vi "savenload.vi"() -> (3 "load error":bool)   [LabVIEW 2012]
uses:
  G_DATA.vi
  G_VEH.vi
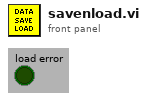
[diagram p1: front panel]
types:
  T1 = enum16{"open", "replace", "create", "open or create", "replace or create", "replace or create with confirmation"}
  T2 = cluster{"M6006":string, "M7042":string, "Tcandata":string, "LaserData":string, "SensorData":string, "B_Sencor data 2202":string, "B_object data 2221":string, "Tmobileye":string}
  T3 = cluster{"M6006":string, "M7042":string, "Tcandata":string, "LaserData":string, "SensorData":string, "B_Sencor data 2202":string, "B_object data 2221":string}
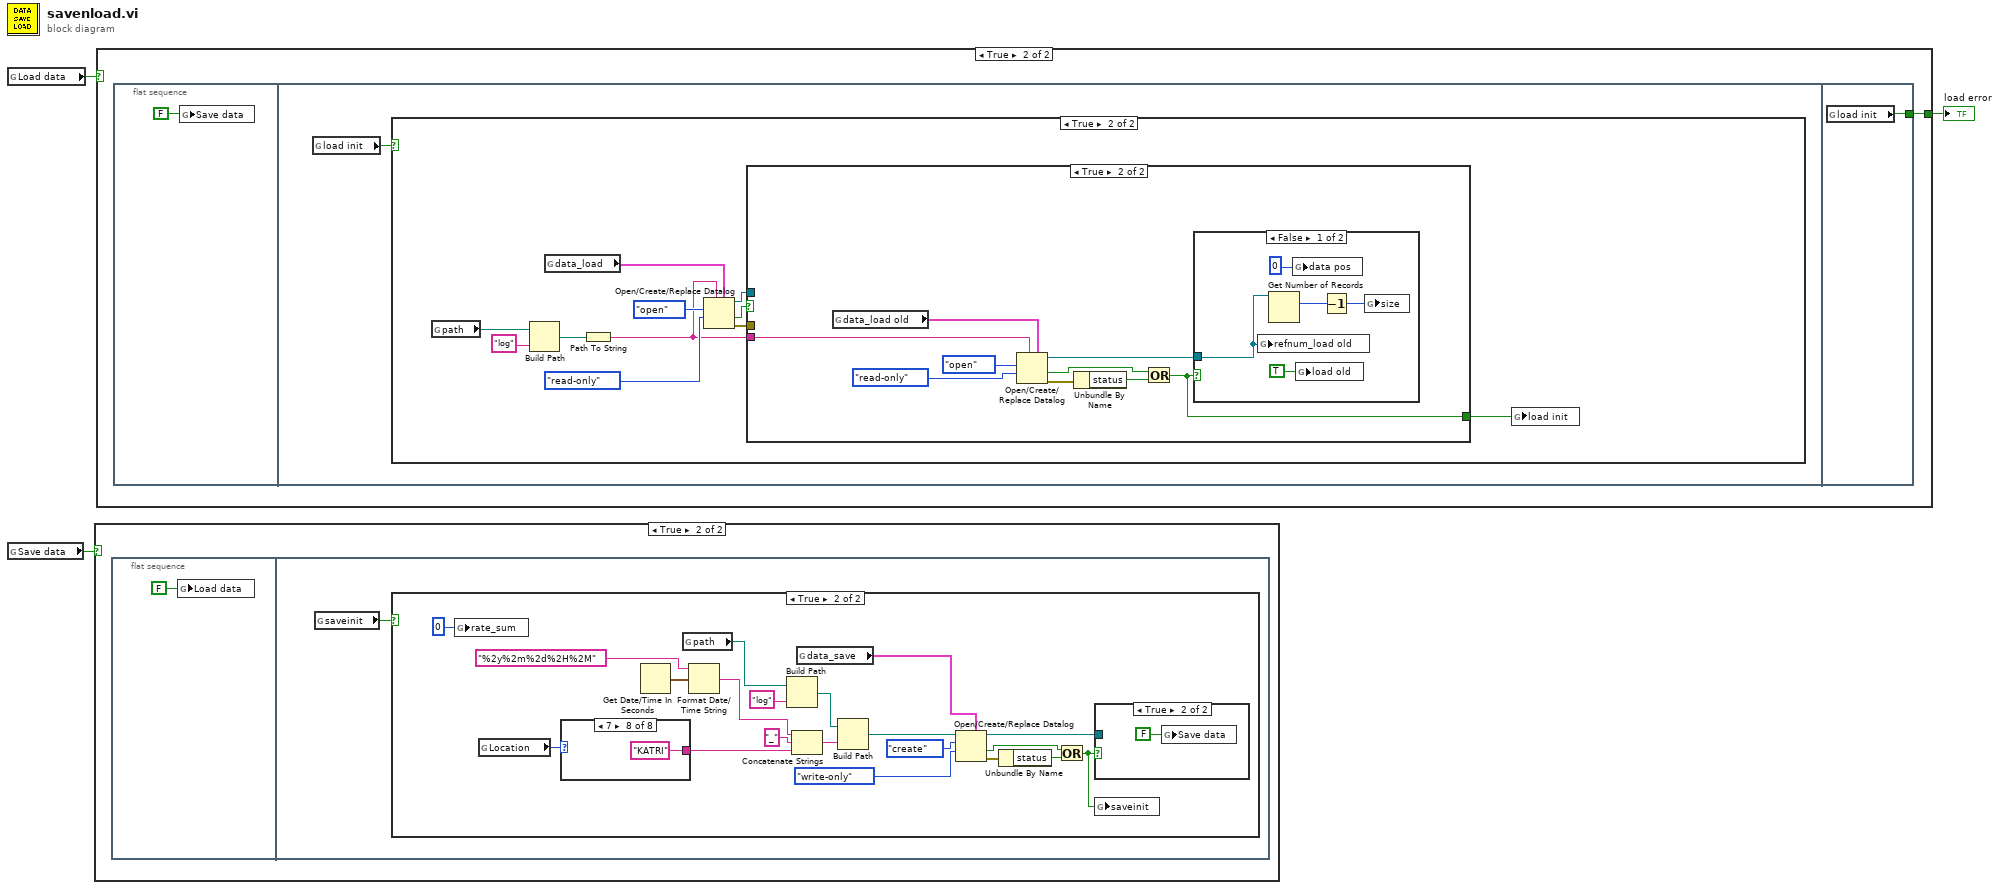
[diagram p0: block diagram]
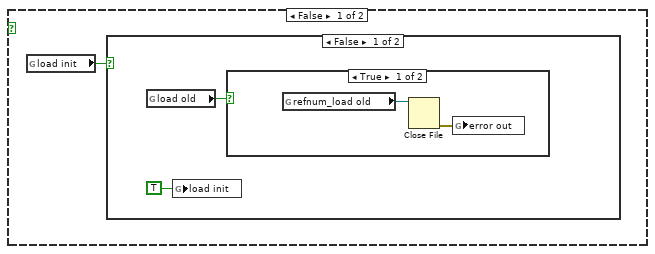
[diagram p2: hidden frame]
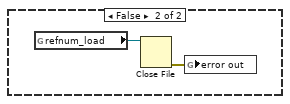
[diagram p3: hidden frame]
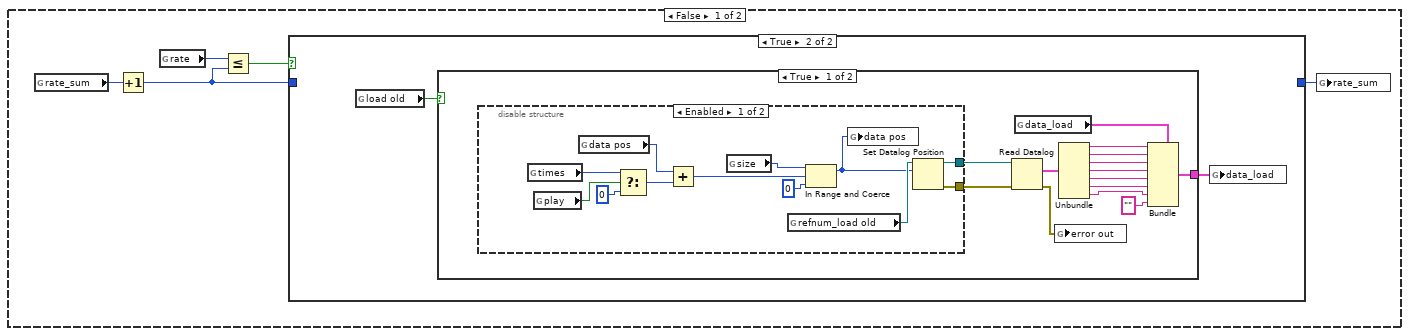
[diagram p5: hidden frame]
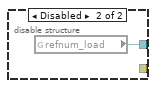
[diagram p7: hidden frame]
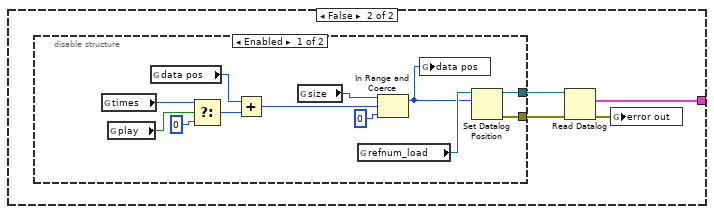
[diagram p8: hidden frame]
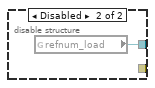
[diagram p9: hidden frame]
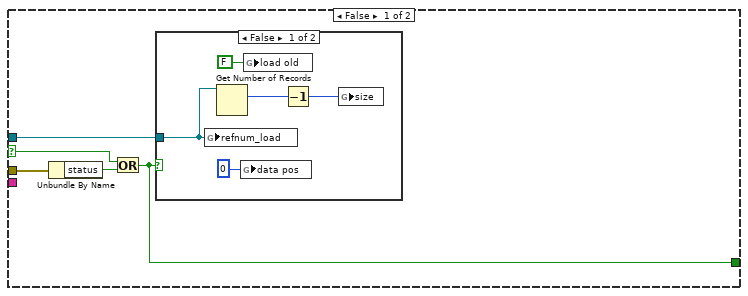
[diagram p10: hidden frame]
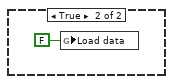
[diagram p11: hidden frame]
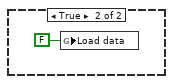
[diagram p12: hidden frame]
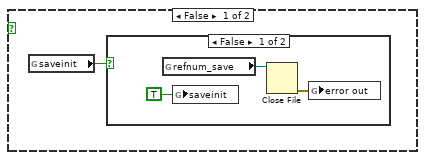
[diagram p13: hidden frame]
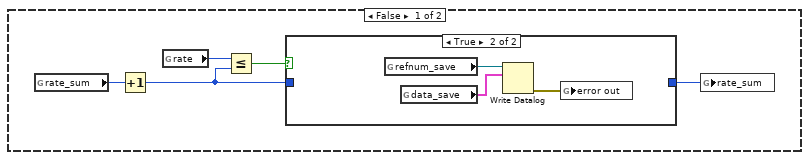
[diagram p15: hidden frame]
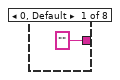
[diagram p17: hidden frame]
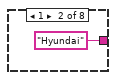
[diagram p18: hidden frame]
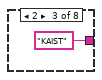
[diagram p19: hidden frame]
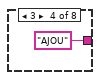
[diagram p20: hidden frame]
diagram:
  n1 = global read "G_DATA.vi" "Load data"() -> (w1:bool)
  n2 = global read "G_DATA.vi" "Save data"() -> (w3:bool)
  n3 = case shown="True" w3 {
    frame False {
      n4 = global read "G_DATA.vi" "saveinit"() -> (w4:bool)
      n5 = case shown="False" w4 {
        frame False {
          n6 = global read "G_DATA.vi" "refnum_save"() -> (w7:refnum<k1>)
          n7 = global write "G_DATA.vi" "saveinit"(TRUE ("saveinit")) -> ()
          n8 = Close File(refnum=w7) -> (error out=w5:errorcluster)  [unwired: 1 in, 1 out]
          n9 = global write "G_DATA.vi" "error out"(w5) -> ()
        }
        frame True {
        }
      }
    }
    frame True {
      n10 = flat-sequence {
        frame #0 {
          n11 = global write "G_DATA.vi" "Load data"(FALSE ("Visible")) -> ()
        }
        frame #1 {
          n12 = global read "G_DATA.vi" "saveinit"() -> (w9:bool)
          n13 = case shown="True" w9 {
            frame False {
              n14 = global read "G_DATA.vi" "rate_sum"() -> (w14:u8)
              n15 = Increment(x=w14) -> (x+1=w10:u8)
              n16 = global read "G_DATA.vi" "rate"() -> (w11:u8)
              n17 = Less Or Equal?(x=w11, y=w10) -> (x <= y?=w13:bool)
              n18 = case shown="True" w13 {
                tunnel: [w15 _] -> w12
                tunnel: w10 -> [w15 _]
                frame False {
                }
                frame True {
                  n19 = global read "G_DATA.vi" "refnum_save"() -> (w18:refnum<k1>)
                  n20 = global read "G_DATA.vi" "data_save"() -> (w17:T2)
                  n21 = Write Datalog(6:w17, 7:w18) -> (0:w16:errorcluster)  [unwired: 1 in, 1 out]
                  n22 = global write "G_DATA.vi" "error out"(w16) -> ()
                }
              }
              n23 = global write "G_DATA.vi" "rate_sum"(w12) -> ()
            }
            frame True {
              n24 = global write "G_DATA.vi" "rate_sum"(u8 0 ("rate_sum")) -> ()
              n25 = global read "G_VEH.vi" "Location"() -> (w29:i32)
              n26 = case shown="7" w29 {
                tunnel: ["" ("String") "Hyundai" ("String") "KAIST" ("String") "AJOU" ("String") "MUNJI" ("String") "Airforce" ("String") "CAR" ("String") "KATRI" ("String")] -> w28
                frame 0, Default {
                }
                frame 1 {
                }
                frame 2 {
                }
                frame 3 {
                }
                frame 4 {
                }
                frame 5 {
                }
                frame 6 {
                }
                frame 7 {
                }
              }
              n27 = Get Date/Time In Seconds() -> (seconds since 1Jan1904=w32:timestamp)
              n28 = global read "G_DATA.vi" "path"() -> (w20:path)
              n29 = Format Date/Time String(time format string (%c)="%2y%2m%2d%2H%2M", seconds (now)=w32) -> (date/time string=w26:string)  [unwired: 1 in]
              n30 = Build Path(base path=w20, name or relative path="log") -> (appended path=w19:path)
              n31 = Concatenate Strings(w26, "_" ("string"), w28) -> (w25:string)
              n32 = global read "G_DATA.vi" "data_save"() -> (w35:T2)
              n33 = Build Path(base path=w19, name or relative path=w25) -> (appended path=w30:path)
              n34 = Open/Create/Replace Datalog(5:w35, 9:enum16{"read/write", "read-only", "write-only"}."write-only" ("access (0:read/write)"), 10:T1."create" ("operation (0:open)"), 11:w30) -> (0:w36:errorcluster, 1:w24:bool, 3:w34:refnum<k1>)  [unwired: 1 in, 1 out]
              n35 = Unbundle By Name(w36) -> ("status"=w23:bool)
              n36 = Or(x=w24, y=w23) -> (x .or. y?=w22:bool)
              n37 = case shown="True" w22 {
                tunnel: w34 -> [w47 _]
                frame False {
                  n38 = global write "G_DATA.vi" "refnum_save"(w47) -> ()
                }
                frame True {
                  n39 = global write "G_DATA.vi" "Save data"(FALSE ("Save data")) -> ()
                }
              }
              n40 = global write "G_DATA.vi" "saveinit"(w22) -> ()
            }
          }
        }
      }
    }
  }
  n41 = case shown="True" w1 {
    tunnel: [_ w56] -> w2
    frame False {
      n42 = global read "G_DATA.vi" "load init"() -> (w49:bool)
      n43 = case shown="False" w49 {
        frame False {
          n44 = global read "G_DATA.vi" "load old"() -> (w50:bool)
          n45 = global write "G_DATA.vi" "load init"(TRUE ("saveinit")) -> ()
          n46 = case shown="True" w50 {
            frame True {
              n47 = global read "G_DATA.vi" "refnum_load old"() -> (w52:refnum<k1>)
              n48 = Close File(refnum=w52) -> (error out=w53:errorcluster)  [unwired: 1 in, 1 out]
              n49 = global write "G_DATA.vi" "error out"(w53) -> ()
            }
            frame False {
              n50 = global read "G_DATA.vi" "refnum_load"() -> (w54:refnum<k1>)
              n51 = Close File(refnum=w54) -> (error out=w55:errorcluster)  [unwired: 1 in, 1 out]
              n52 = global write "G_DATA.vi" "error out"(w55) -> ()
            }
          }
        }
        frame True {
        }
      }
    }
    frame True {
      n53 = flat-sequence {
        tunnel: [w148] -> w56
        frame #0 {
          n54 = global write "G_DATA.vi" "Save data"(FALSE ("Save data")) -> ()
        }
        frame #1 {
          n55 = global read "G_DATA.vi" "load init"() -> (w58:bool)
          n56 = case shown="True" w58 {
            frame False {
              n57 = global read "G_DATA.vi" "rate_sum"() -> (w62:u8)
              n58 = Increment(x=w62) -> (x+1=w59:u8)
              n59 = global read "G_DATA.vi" "rate"() -> (w63:u8)
              n60 = Less Or Equal?(x=w63, y=w59) -> (x <= y?=w61:bool)
              n61 = case shown="True" w61 {
                tunnel: [w64 _] -> w60
                tunnel: w59 -> [w64 _]
                frame False {
                }
                frame True {
                  n62 = global read "G_DATA.vi" "load old"() -> (w66:bool)
                  n63 = case shown="True" w66 {
                    tunnel: [w70 w94] -> w65
                    frame True {
                      n64 = disable-structure shown="Enabled" {
                        disable-tunnel: [w84 _] -> w80
                        disable-tunnel: [w83 w93] -> w78
                        frame Enabled {
                          n65 = global read "G_DATA.vi" "times"() -> (w89:i64)
                          n66 = global read "G_DATA.vi" "play"() -> (w90:bool)
                          n67 = global read "G_DATA.vi" "data pos"() -> (w92:i64)
                          n68 = Select(t=w89, s=w90, f=i64 0) -> (s? t:f=w85:i64)
                          n69 = Add(x=w92, y=w85) -> (x+y=w87:i64)
                          n70 = global read "G_DATA.vi" "size"() -> (w91:i64)
                          n71 = global read "G_DATA.vi" "refnum_load old"() -> (w82:refnum<k1>)
                          n72 = In Range and Coerce(upper limit=w91, x=w87, lower limit=i64 0) -> (coerced(x)=w81:i64)  [unwired: 1 out]
                          n73 = global write "G_DATA.vi" "data pos"(w81) -> ()
                          n74 = Set Datalog Position(6:w81, 7:w82) -> (0:w84:errorcluster, 3:w83:refnum<k1>)  [unwired: 2 in]
                        }
                        frame Disabled {
                          n75 = global read "G_DATA.vi" "refnum_load"() -> (w93:refnum<k1>)
                        }
                      }
                      n76 = Read Datalog(4:w80, 7:w78) -> (0:w79:errorcluster, 2:w77:T3)  [unwired: 2 out]
                      n77 = global read "G_DATA.vi" "data_load"() -> (w71:T2)
                      n78 = global write "G_DATA.vi" "error out"(w79) -> ()
                      n79 = Unbundle(w77) -> ("M6006"=w76:string, "M7042"=w75:string, "Tcandata"=w74:string, "LaserData"=w73:string, "SensorData"=w72:string, "B_Sencor data 2202"=w69:string, "B_object data 2221"=w68:string)
                      n80 = Bundle(cluster=w71, "M6006"=w76, "M7042"=w75, "Tcandata"=w74, "LaserData"=w73, "SensorData"=w72, "B_Sencor data 2202"=w69, "B_object data 2221"=w68, "Tmobileye"="" ("B_Sencor data 2202")) -> (w70:T2)
                    }
                    frame False {
                      n81 = disable-structure shown="Enabled" {
                        disable-tunnel: [w101 _] -> w97
                        disable-tunnel: [w100 w110] -> w95
                        frame Enabled {
                          n82 = global read "G_DATA.vi" "times"() -> (w106:i64)
                          n83 = global read "G_DATA.vi" "play"() -> (w107:bool)
                          n84 = global read "G_DATA.vi" "data pos"() -> (w109:i64)
                          n85 = Select(t=w106, s=w107, f=i64 0) -> (s? t:f=w102:i64)
                          n86 = Add(x=w109, y=w102) -> (x+y=w104:i64)
                          n87 = global read "G_DATA.vi" "size"() -> (w108:i64)
                          n88 = global read "G_DATA.vi" "refnum_load"() -> (w99:refnum<k1>)
                          n89 = In Range and Coerce(upper limit=w108, x=w104, lower limit=i64 0) -> (coerced(x)=w98:i64)  [unwired: 1 out]
                          n90 = global write "G_DATA.vi" "data pos"(w98) -> ()
                          n91 = Set Datalog Position(6:w98, 7:w99) -> (0:w101:errorcluster, 3:w100:refnum<k1>)  [unwired: 2 in]
                        }
                        frame Disabled {
                          n92 = global read "G_DATA.vi" "refnum_load"() -> (w110:refnum<k1>)
                        }
                      }
                      n93 = Read Datalog(4:w97, 7:w95) -> (0:w96:errorcluster, 2:w94:T2)  [unwired: 2 out]
                      n94 = global write "G_DATA.vi" "error out"(w96) -> ()
                    }
                  }
                  n95 = global write "G_DATA.vi" "data_load"(w65) -> ()
                }
              }
              n96 = global write "G_DATA.vi" "rate_sum"(w60) -> ()
            }
            frame True {
              n97 = global read "G_DATA.vi" "path"() -> (w114:path)
              n98 = Build Path(base path=w114, name or relative path="log") -> (appended path=w112:path)
              n99 = global read "G_DATA.vi" "data_load"() -> (w119:T2)
              n100 = Path To String(path=w112) -> (string=w111:string)
              n101 = Open/Create/Replace Datalog(5:w119, 7:w111, 9:enum16{"read/write", "read-only", "write-only"}."read-only" ("access (0:read/write)"), 10:T1."open" ("operation (0:open)")) -> (0:w117:errorcluster, 1:w118:bool, 3:w116:refnum<k1>)  [unwired: 2 in]
              n102 = case shown="True" w118 {
                selector: w118 -> [w125 _]
                tunnel: w117 -> [w124 _]
                tunnel: w116 -> [w123 _]
                tunnel: [w122 w134] -> w115
                tunnel: w111 -> [_ w133]
                frame False {
                  n103 = Unbundle By Name(w124) -> ("status"=w126:bool)
                  n104 = Or(x=w125, y=w126) -> (x .or. y?=w122:bool)
                  n105 = case shown="False" w122 {
                    tunnel: w123 -> [w129 _]
                    frame False {
                      n106 = global write "G_DATA.vi" "refnum_load"(w129) -> ()
                      n107 = Get Number of Records(7:w129) -> (2:w130:i64)  [unwired: 1 in, 2 out]
                      n108 = global write "G_DATA.vi" "data pos"(i64 0 ("data pos")) -> ()
                      n109 = global write "G_DATA.vi" "load old"(FALSE ("load old")) -> ()
                      n110 = Decrement(x=w130) -> (x-1=w131:i64)
                      n111 = global write "G_DATA.vi" "size"(w131) -> ()
                    }
                    frame True {
                      n112 = global write "G_DATA.vi" "Load data"(FALSE ("Save data")) -> ()
                    }
                  }
                }
                frame True {
                  n113 = global read "G_DATA.vi" "data_load old"() -> (w141:T3)
                  n114 = Open/Create/Replace Datalog(5:w141, 7:w133, 9:enum16{"read/write", "read-only", "write-only"}."read-only" ("access (0:read/write)"), 10:T1."open" ("operation (0:open)")) -> (0:w137:errorcluster, 1:w136:bool, 3:w135:refnum<k1>)  [unwired: 2 in]
                  n115 = Unbundle By Name(w137) -> ("status"=w138:bool)
                  n116 = Or(x=w136, y=w138) -> (x .or. y?=w134:bool)
                  n117 = case shown="False" w134 {
                    tunnel: w135 -> [w144 _]
                    frame False {
                      n118 = global write "G_DATA.vi" "refnum_load old"(w144) -> ()
                      n119 = Get Number of Records(7:w144) -> (2:w145:i64)  [unwired: 1 in, 2 out]
                      n120 = global write "G_DATA.vi" "data pos"(i64 0 ("data pos")) -> ()
                      n121 = global write "G_DATA.vi" "load old"(TRUE ("load old")) -> ()
                      n122 = Decrement(x=w145) -> (x-1=w146:i64)
                      n123 = global write "G_DATA.vi" "size"(w146) -> ()
                    }
                    frame True {
                      n124 = global write "G_DATA.vi" "Load data"(FALSE ("Save data")) -> ()
                    }
                  }
                }
              }
              n125 = global write "G_DATA.vi" "load init"(w115) -> ()
            }
          }
        }
        frame #2 {
          n126 = global read "G_DATA.vi" "load init"() -> (w148:bool)
        }
      }
    }
  }
  "load error" <- w2
